vi "Dialogue Window.vi"(7 "Colour":u32(colorbox)=16777225, 8 "error in (no error)":errorcluster, 9 "Caption-Left button (Cancel)":string, 10 "Caption-Right button (OK)":string, 11 "Message string":string) -> (0 "error out":errorcluster, 1 "Cancelled (Left button pressed)":bool, 3 "Panel closed":bool)   [LabVIEW 2013]
doc: "Use this template to create a dialog box with event handling."
uses:
  <vilib>/Utility/miscctls.llb/LVPointTypeDef.ctl
  Global Variables/General Globals.vi
panel:
  in  "Left Button":bool
  in  "Rigth Button":bool
  out "Message":string
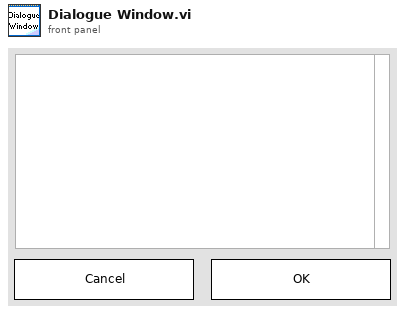
[diagram p1: front panel]
types:
  T1 = typedef "LVPointTypeDef.ctl" = cluster{"Horizontal":i16, "Vertical":i16}
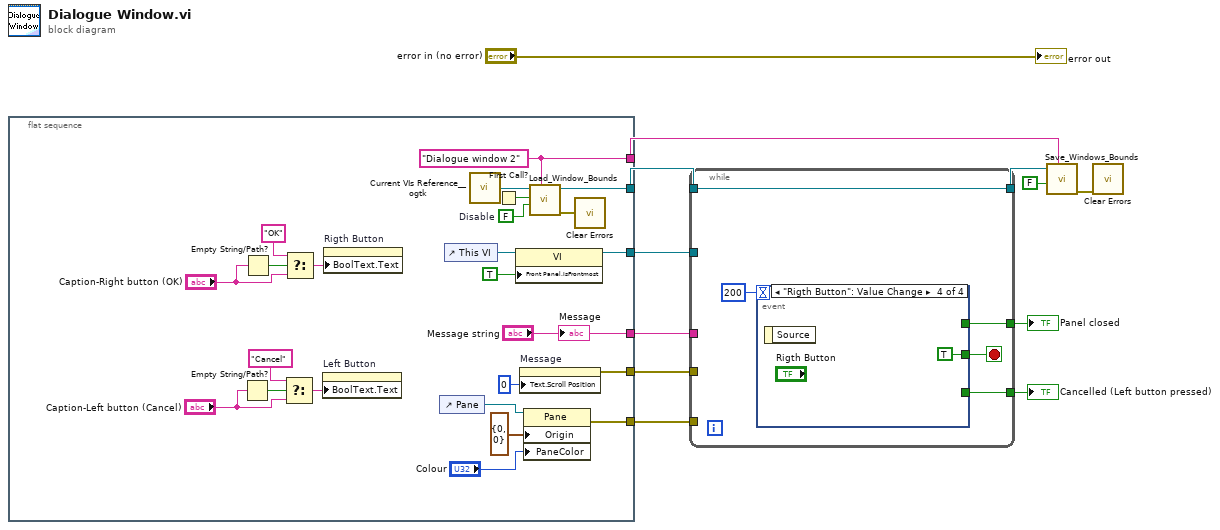
[diagram p0: block diagram]
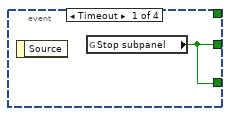
[diagram p2: hidden frame]
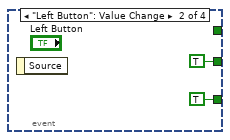
[diagram p3: hidden frame]
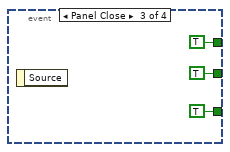
[diagram p4: hidden frame]
diagram:
  n1 = flat-sequence {
    tunnel: ["Message string"] -> w12
    tunnel: [w34] -> w11
    tunnel: [w31] -> w10
    tunnel: [w29] -> w9
    tunnel: [w24] -> w7
    tunnel: [w23] -> w5
    frame #0 {
      w25 = FALSE  # Disable
      w24 = "Dialogue window 2" ("Window Name (i.e. Key)")
      n2 = Empty String/Path?(string/path="Caption-Left button (Cancel)") -> (empty?=w17:bool)
      n3 = Empty String/Path?(string/path="Caption-Right button (OK)") -> (empty?=w21:bool)
      n4 = Select(t="Cancel", s=w17, f="Caption-Left button (Cancel)") -> (s? t:f=w16:string)
      n5 = Select(t="OK", s=w21, f="Caption-Right button (OK)") -> (s? t:f=w19:string)
      n6 = property on="Left Button" class="Bool"("BoolText.Text"=w16) -> ()  [unwired: 2 in, 2 out]
      n7 = property on="Rigth Button" class="Bool"("BoolText.Text"=w19) -> ()  [unwired: 2 in, 2 out]
      n8 = control-ref of="Pane"() -> (w28:refnum<vi>)
      n9 = control-ref of="This VI"() -> (w32:refnum<vi>)
      n10 = call "Current VIs Reference__ogtk.vi"() -> ("Current VI's reference"=w27:refnum<vi>)  [unwired: 5 in]
      n11 = First Call?() -> (First Call?: T/F=w26:bool)
      n12 = property on="Property Node" class="VI"(reference=w32, "Front Panel.IsFrontmost"=TRUE ("Front Panel Window:Is Frontmost")) -> (reference out=w31:refnum<vi>)  [unwired: 1 in, 1 out]
      n13 = property on="Message" class="Str"("Text.Scroll Position"=u32 0) -> (error out=w34:errorcluster)  [unwired: 2 in, 1 out]
      n14 = property class="Pane"(reference=w28, "Origin"=T1 {"Horizontal"=0, "Vertical"=0}, "PaneColor"="Colour") -> (error out=w29:errorcluster)  [unwired: 1 in, 1 out]
      n15 = call "Load_Window_Bounds.vi"("Window Name (i.e. Key)"=w24, "Disable"=w25, "First Call"=w26, "Window VI's Ref"=w27) -> ("error out"=w13:errorcluster, "reference out"=w23:refnum<vi>)  [unwired: 4 in, 2 out]
      n16 = call <vilib>:"Clear Errors.vi"("error in (no error)"=w13) -> ()  [unwired: 6 in, 1 out]
      "Message" <- "Message string"
    }
  }
  n17 = while {
    tunnel: w12 -> [_]
    tunnel: w11 -> [_]
    tunnel: w9 -> [_]
    tunnel: w10 -> [_]
    tunnel: [w39] -> w8
    tunnel: w5 -> [w38]
    tunnel: [w38] -> w4
    tunnel: [w37] -> w2
    stop <- w41 stop-if-true
    n18 = event shown="[3] \"Rigth Button\": Value Change" {
      selector: _ -> [_ _ _ _]
      dyn-events: _ -> [_ _ _ _]
      timeout: 200 -> [_ _ _ _]
      tunnel: [w42 TRUE ("Stop?") TRUE ("Stop?") TRUE ("Stop?")] -> w41
      tunnel: [w42 TRUE ("Stop subpanel") TRUE ("Stop subpanel") _] -> w39
      tunnel: [_ _ TRUE ("Stop subpanel") _] -> w37
      event Timeout {
        n19 = event-data() -> ()  [unwired: 1 in, 1 out]
        n20 = global read "General Globals.vi" "Stop subpanel"() -> (w42:bool)
      }
      event "Left Button": Value Change {
        n21 = event-data() -> ()  [unwired: 1 in, 1 out]
      }
      event Panel Close {
        n22 = event-data() -> ()  [unwired: 1 in, 1 out]
      }
      event "Rigth Button": Value Change {
        n23 = event-data() -> ()  [unwired: 1 in, 1 out]
      }
    }
  }
  "Cancelled (Left button pressed)" <- w8
  "Panel closed" <- w2
  n24 = call "Save_Windows_Bounds.vi"("Window Name (i.e. Key)"=w7, "Front Panel Window:Open"=FALSE, "Window VI's Ref"=w4) -> ("Error out (pass-through)"=w1:errorcluster)  [unwired: 8 in]
  n25 = call <vilib>:"Clear Errors.vi"("error in (no error)"=w1) -> ()  [unwired: 6 in, 1 out]
  "error out" <- "error in (no error)"
